vi "Write Top caller.vi"(8 "error in (no error)":errorcluster, 10 "Top caller":bool, 11 "Mag Lab Measure Base in":refnum<class "Mag Lab Measure Base.lvclass">) -> (0 "error out":errorcluster, 3 "Mag Lab Measure Base out":refnum<class "Mag Lab Measure Base.lvclass">)   [LabVIEW 2015, in "Mag Lab Measure Base.lvclass"]
uses:
  Mag Lab Measure Base.lvclass
  Mag Lab Measure Base.lvclass/Mag Lab Measure Base.ctl
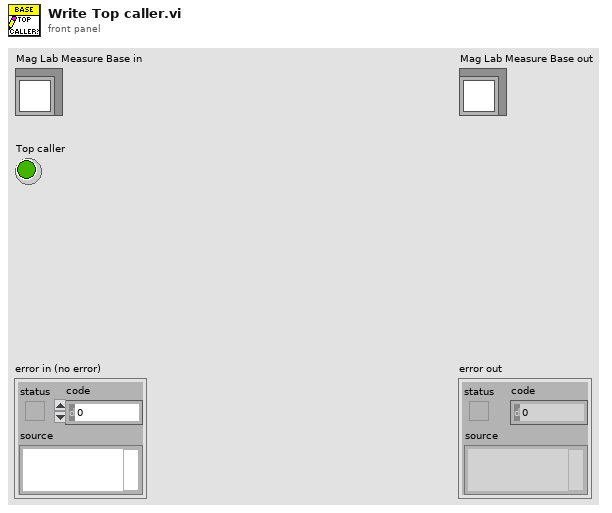
[diagram p1: front panel]
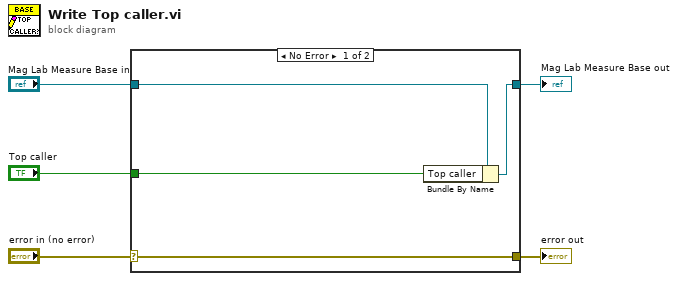
[diagram p0: block diagram]
diagram:
  n1 = case shown="No Error" "error in (no error)" {
    selector: "error in (no error)" -> [w9 w10]
    tunnel: [w9 w10] -> w4
    tunnel: [w7 w11] -> w2
    tunnel: "Mag Lab Measure Base in" -> [w8 w11]
    tunnel: "Top caller" -> [w6 _]
    frame No Error {
      n2 = Bundle By Name(cluster=w8, "Top caller"=w6) -> (w7:refnum<class "Mag Lab Measure Base.lvclass">)
    }
    frame Error {
    }
  }
  "error out" <- w4
  "Mag Lab Measure Base out" <- w2
